vi "LAB8A1.vi"() -> ()   [LabVIEW 2018]
panel:
  out "ANSWER":string
  in  "OFF/ON":bool
  in  "#2":dbl
  in  "#1":dbl
  in  "FUNCTION":dbl(slide) scale=0.0..3.0
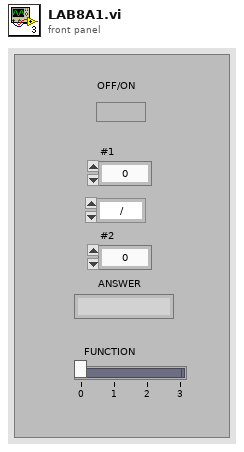
[diagram p1: front panel]
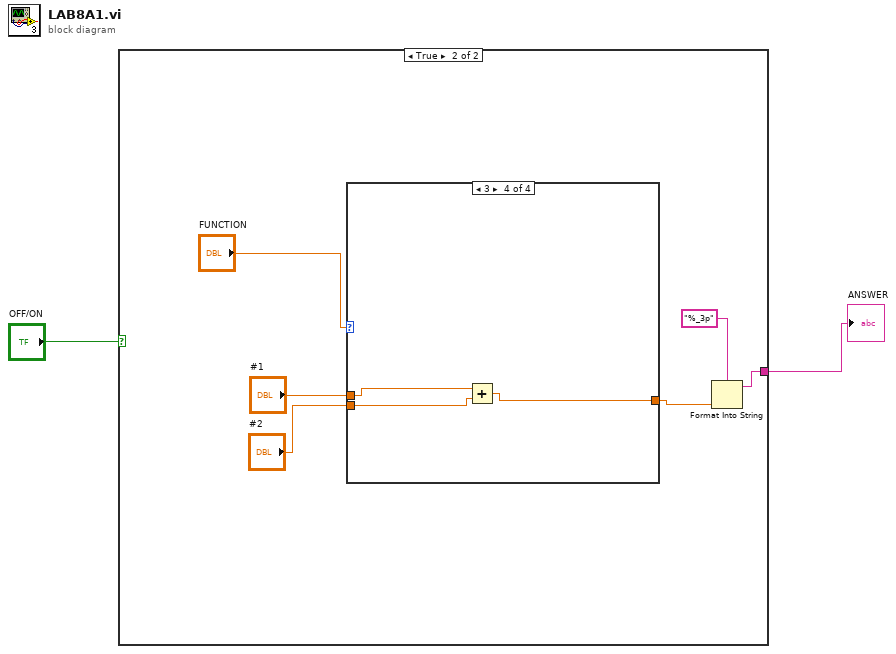
[diagram p0: block diagram]
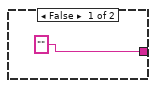
[diagram p2: hidden frame]
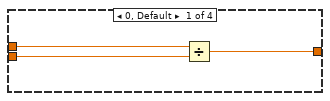
[diagram p3: hidden frame]
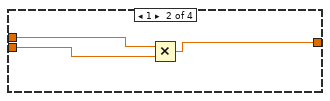
[diagram p4: hidden frame]
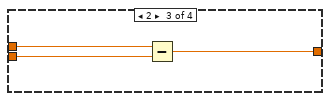
[diagram p5: hidden frame]
diagram:
  n1 = case shown="True" "OFF/ON" {
    tunnel: ["" w5] -> w1
    frame False {
    }
    frame True {
      n2 = case shown="3" "FUNCTION" {
        tunnel: "#1" -> [w12 w15 w18 w21]
        tunnel: "#2" -> [w11 w14 w17 w20]
        tunnel: [w10 w13 w16 w19] -> w6
        frame 0, Default {
          n3 = Divide(x=w12, y=w11) -> (x/y=w10:dbl)
        }
        frame 1 {
          n4 = Multiply(x=w15, y=w14) -> (x*y=w13:dbl)
        }
        frame 2 {
          n5 = Subtract(x=w18, y=w17) -> (x-y=w16:dbl)
        }
        frame 3 {
          n6 = Add(x=w21, y=w20) -> (x+y=w19:dbl)
        }
      }
      n7 = Format Into String(format string="%_3p", w6) -> (resulting string=w5:string)  [unwired: 2 in, 1 out]
    }
  }
  "ANSWER" <- w1
